vi "ITickable Tick.vi"(8 "error in (no error)":errorcluster, 11 "Snake in":refnum<class "Snake.lvclass">) -> (0 "error out":errorcluster, 3 "Snake out":refnum<class "Snake.lvclass">)   [LabVIEW 2020, in "Snake.lvclass"]
uses:
  Snake.lvclass
  Snake.lvclass/Snake.ctl
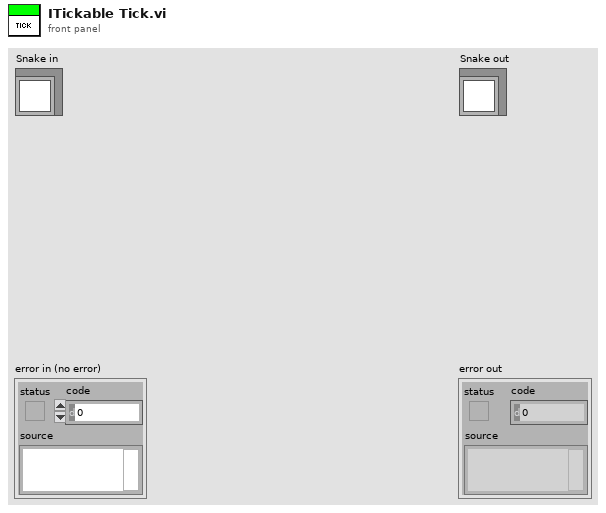
[diagram p1: front panel]
types:
  T1 = typedef "Snake.lvclass/Snake Segment STYP.ctl" = cluster{"Location":cluster{"x":u32, "y":u32}, "Direction":T2}
  T2 = typedef "Direction STYP.ctl" = enum16{"Up", "Down", "Left", "Right"}
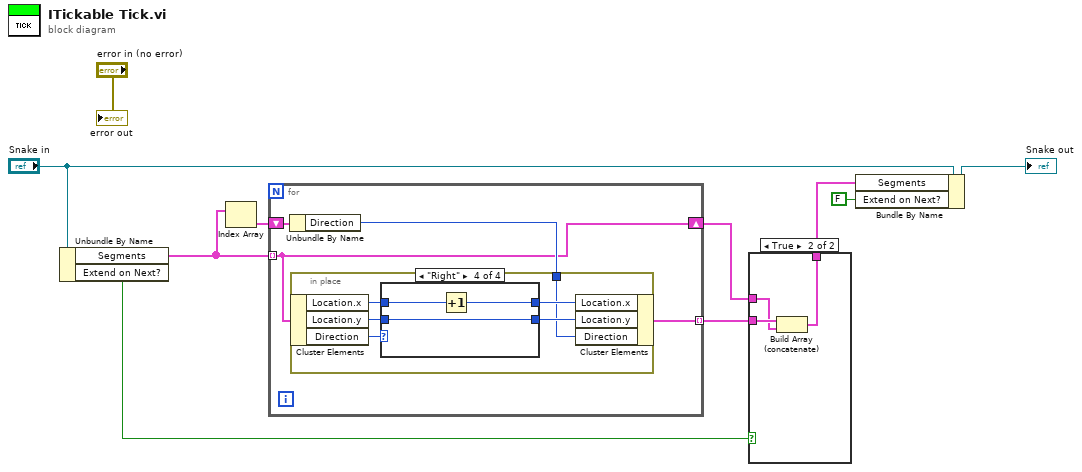
[diagram p0: block diagram]
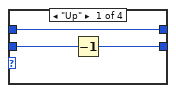
[diagram p3: hidden frame]
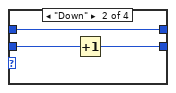
[diagram p4: hidden frame]
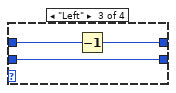
[diagram p5: hidden frame]
diagram:
  n1 = Unbundle By Name("Snake in") -> ("Segments"=w8:T1[], "Extend on Next?"=w5:bool)
  n2 = Index Array(array=w8) -> (element=w9:T1)  [unwired: 1 in]
  n3 = for {
    tunnel: w8 -> [w11] mode=indexing
    shift-right: [w11] -> w2
    shift-left: w9 -> [w14]
    tunnel: [w12] -> w4 mode=indexing
    n4 = Unbundle By Name(w14) -> ("Direction"=w13:T2)
    n5 = in-place {
      in-place-border: w13 -> [w15]
      n6 = in-place-cluster #1(w11) -> ("Location.x"=w19:u32, "Location.y"=w18:u32, "Direction"=w20:T2)
      n7 = case shown="\"Right\"" w20 {
        tunnel: w19 -> [w23 w26 w29 w32]
        tunnel: w18 -> [w22 w25 w28 w31]
        tunnel: [w23 w26 w27 w30] -> w17
        tunnel: [w21 w24 w28 w31] -> w16
        frame "Up" {
          n8 = Decrement(x=w22) -> (x-1=w21:u32)
        }
        frame "Down" {
          n9 = Increment(x=w25) -> (x+1=w24:u32)
        }
        frame "Left" {
          n10 = Decrement(x=w29) -> (x-1=w27:u32)
        }
        frame "Right" {
          n11 = Increment(x=w32) -> (x+1=w30:u32)
        }
      }
      n12 = in-place-cluster #1("Location.x"=w17, "Location.y"=w16, "Direction"=w15) -> (w12:T1)
    }
  }
  n13 = case shown="True" w5 {
    tunnel: w4 -> [w33 w36]
    tunnel: [w33 w34] -> w3
    tunnel: w2 -> [_ w35]
    frame False {
    }
    frame True {
      n14 = Build Array (concatenate)(w36, w35) -> (w34:T1[])
    }
  }
  n15 = Bundle By Name(cluster="Snake in", "Segments"=w3, "Extend on Next?"=FALSE) -> (→"Snake out":refnum<class "Snake.lvclass">)
  "error out" <- "error in (no error)"
